vi "Test.vi"   [LabVIEW 2014]
doc: "This VI is called when test mode begins, and will automatically be terminated when it ends. You can add manual or automatic tests and invoke them from the dashboard."
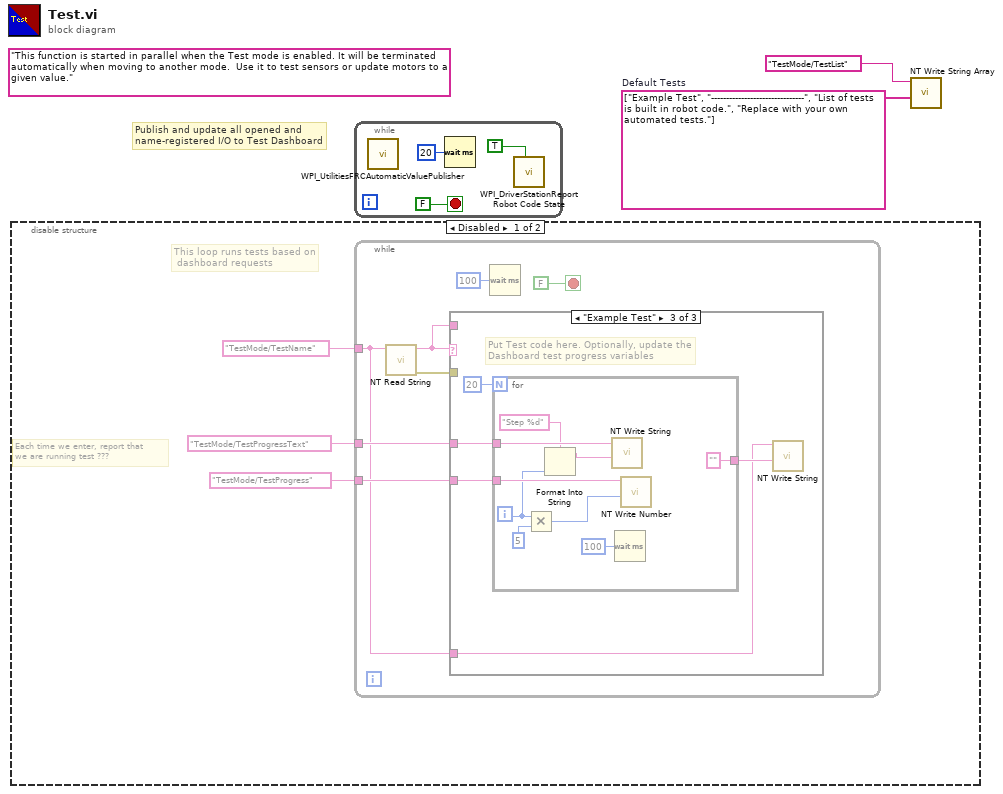
[diagram p0: block diagram]
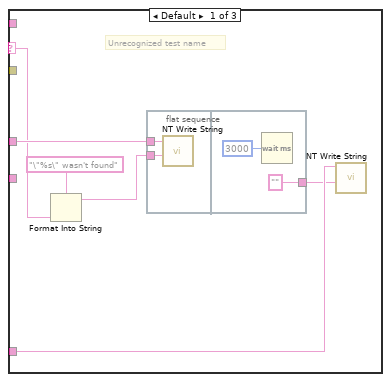
[diagram p2: hidden frame]
diagram:
  w2 = string[] ["Example Test", "-------------------------------", "List of tests is built in robot code.", "Replace with your own automated tests."]  # Default Tests
  (unwired) "This function is started in parallel when the Test mode is enabled. It will be terminated automatically when moving to another mode.  Use it to test sensors or update motors to a given value."
  # "Publish and update all opened and\nname-registered I/O to Test Dashboard"
  n1 = disable-structure shown="Disabled" {
    frame Disabled {
      # "This loop runs tests based on \n dashboard requests"
      # "Each time we enter, report that\nwe are running test ???"
      n2 = while {
        tunnel: "TestMode/TestName" ("Name") -> [w7]
        tunnel: "TestMode/TestProgressText" ("Name") -> [w10]
        tunnel: "TestMode/TestProgress" ("Name") -> [w9]
        stop <- FALSE stop-if-true
        n3 = call <vilib>:"NT Read String.vi"("Name"=w7) -> ("error out"=w6:errorcluster, "String"=w8:string)  [unwired: 9 in]
        n4 = case shown="\"Example Test\"" w8 {
          selector: w8 -> [w17 _ _]
          tunnel: w7 -> [w14 _ w23]
          tunnel: w10 -> [w18 _ w26]
          tunnel: w9 -> [_ _ w27]
          tunnel: w8 -> [_ _ _]
          tunnel: w6 -> [_ _ _]
          frame Default {
            # "Unrecognized test name"
            n5 = Format Into String(format string="\"%s\" wasn't found" ("Name"), w17) -> (resulting string=w16:string)  [unwired: 2 in, 1 out]
            n6 = flat-sequence {
              tunnel: w18 -> [w19]
              tunnel: w16 -> [w20]
              tunnel: ["" ("Name")] -> w13
              frame #0 {
                n7 = call <vilib>:"NT Write String.vi"("String"=w20, "Name"=w19) -> ()  [unwired: 9 in, 1 out]
              }
              frame #1 {
                n8 = Wait (ms)(milliseconds to wait=u32 3000) -> ()  [unwired: 1 out]
              }
            }
            n9 = call <vilib>:"NT Write String.vi"("String"=w13, "Name"=w14) -> ()  [unwired: 9 in, 1 out]
          }
          frame "" {
            # "No test to run"
          }
          frame "Example Test" {
            # "Put Test code here. Optionally, update the\nDashboard test progress variables"
            n10 = for {
              N: 20 -> [_]
              tunnel: w27 -> [w36]
              tunnel: w26 -> [w34]
              tunnel: ["" ("String")] -> w24
              i -> [w31]
              n11 = Multiply(x=w31, y=u32 5 ("milliseconds to wait")) -> (x*y=w32:u32)
              n12 = Format Into String(format string="Step %d", w31) -> (resulting string=w29:string)  [unwired: 2 in, 1 out]
              n13 = call <vilib>:"NT Write String.vi"("String"=w29, "Name"=w34) -> ()  [unwired: 9 in, 1 out]
              n14 = Wait (ms)(milliseconds to wait=u32 100) -> ()  [unwired: 1 out]
              n15 = call <vilib>:"NT Write Number.vi"("Numeric"=w32, "Name"=w36) -> ()  [unwired: 9 in, 1 out]
            }
            n16 = call <vilib>:"NT Write String.vi"("String"=w24, "Name"=w23) -> ()  [unwired: 9 in, 1 out]
          }
        }
        n17 = Wait (ms)(milliseconds to wait=u32 100) -> ()  [unwired: 1 out]
      }
    }
    frame Enabled {
    }
  }
  n18 = while {
    stop <- FALSE stop-if-true
    n19 = call <vilib>:"WPI_UtilitiesFRCAutomaticValuePublisher.vi"() -> ()  [unwired: 12 in]
    n20 = Wait (ms)(milliseconds to wait=u32 20) -> ()  [unwired: 1 out]
    n21 = call <vilib>:"WPI_DriverStationReport Robot Code State.vi"("Test"=TRUE ("Autonomous")) -> ()  [unwired: 10 in, 1 out]
  }
  n22 = call <vilib>:"NT Write String Array.vi"("String Array"=w2, "Name"="TestMode/TestList") -> ()  [unwired: 9 in, 1 out]
